vi "子界面-查看某框-不显示界面.vi"(0 "框号":dbl format="%#_13g", 1 "框组":T3(array[cluster]), 2 "临界Z值":i32, 3 "反射图原始路径":path, 4 "临界面积百分比值":dbl, 5 "预先配置的灰度阈值":dbl, 6 "穿透图原始路径":path, 7 "部位信息":string[](array[string])=["", "34.500000", "32.500000", "1121", "34", "54.955926", "分层类", "不合格", ""], 12 "产品规格":cluster{"产品长度（周长）（mm）":dbl, "产品宽度（母线长）（mm）":dbl}) -> (14 "弥散类检测结果":string[][](table), 19 "分层类检测结果":string[][](table))   [LabVIEW 2018]
uses:
  <vilib>/vision/NI_Vision_Development_Module.lvlib
panel:
  out "弥散和分层临界灰度值":i32
  out "弥散缺陷个数":i32
  out "分层缺陷个数":i32
  out "合格？ 弥散类":string="fencengThreshold"
  out "合格？分层类":string="fencengThreshold"
  out "?":T1(plugin-control)
  out "Threshold Image":T1(plugin-control)
  out "Threshold Image":T1(plugin-control)
  out "Threshold Image":T1(plugin-control)
  in  "Tab Control":T2
  out "穿透ROI":T1(plugin-control)
  out "Threshold Image":T1(plugin-control)
  out "?":T1(plugin-control)
  out "?":T1(plugin-control)
  out "Threshold Image":T1(plugin-control)
  out "Threshold Image":T1(plugin-control)
  out "弥散测量结果":dbl[][](array[numeric]) format="%.2f"
  in  "分隔符（'\\'代码显示）":string="\t"
  in  "格式字符串":string="%f"
  out "面积 (pixels)":i32
  in  "格式字符串 2":string="%f"
  in  "分隔符（'\\'代码显示）":string="\t"
  out "分层测量结果":dbl[][](array[numeric]) format="%.2f"
  out "缺陷分类的临界值":sgl format="%#.3f"
  # "所选区域信息"
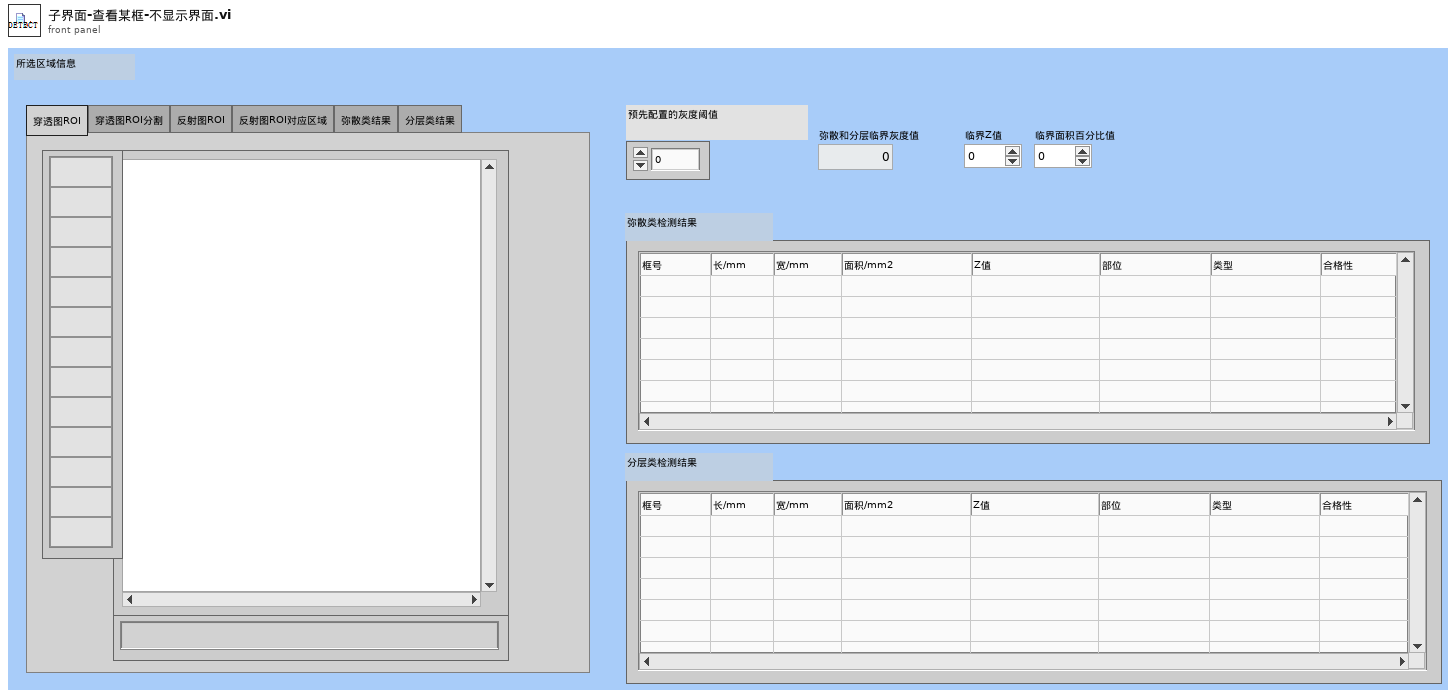
[diagram p1: front panel]
types:
  T1 = typedef "IMAQ Image.ctl" = refnum<image>
  T2 = typedef "控件 1.ctl" = enum32{"穿透图ROI", "穿透图ROI分割", "反射图ROI", "反射图ROI对应区域", "弥散类结果", "分层类结果"}
  T3 = cluster{"Global Rectangle":i32[], "Contours":cluster{"Contour Type":u32, "ROI Type":u32, "Points":i32[]}[]}[]
  T4 = typedef "Image Type" = u32
  T5 = typedef "Particle Parameters" = i32
  T6 = cluster{"Measurement Parameter":T5, "Range Lower Value":dbl, "Range Upper Value":dbl, "Range":bool, "Measurement Type":bool}[]
  T7 = cluster{"Global Rectangle":i32[], "Contours":cluster{"Contour Type":u32, "ROI Type":u32, "Points":i32[]}[]}
  T8 = cluster{"histogram":u32[], "Minimal Value":sgl, "Maximal Value":sgl, "Starting Value":sgl, "Interval Width":sgl, "Mean Value":sgl, "Standard  Variation":sgl, "Area (pixels)":i32}
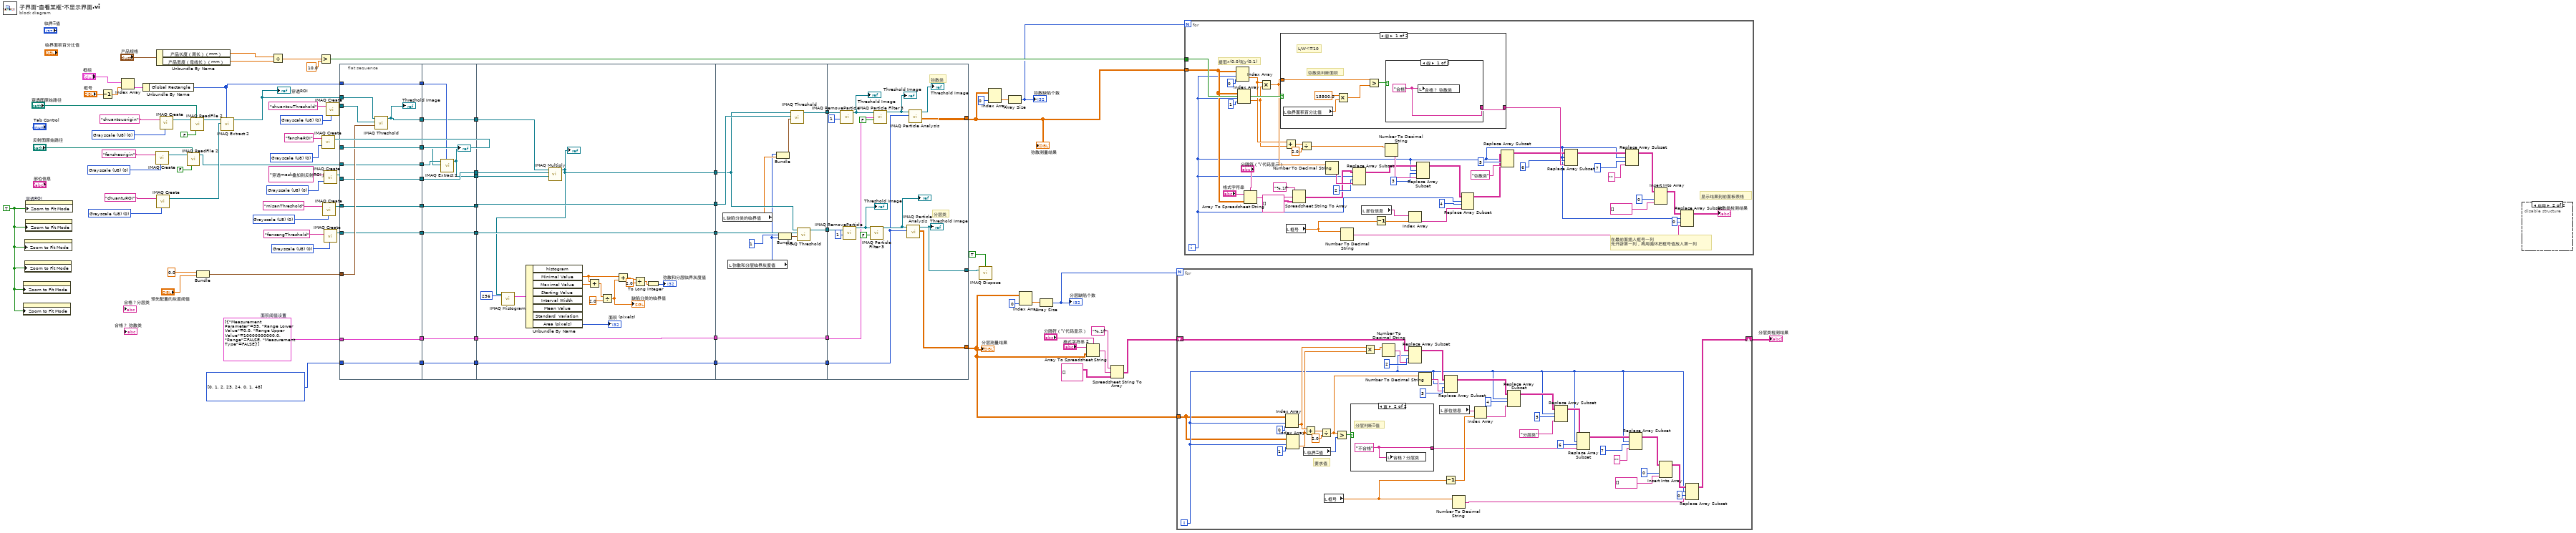
[diagram p0: block diagram]
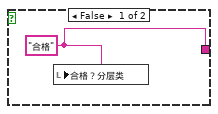
[diagram p2: hidden frame]
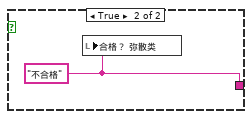
[diagram p3: hidden frame]
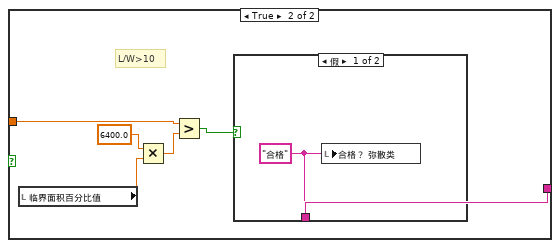
[diagram p4: hidden frame]
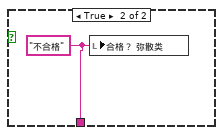
[diagram p5: hidden frame]
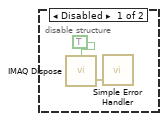
[diagram p6: hidden frame]
diagram:
  w55 = T4 0 items=["Grayscale (U8)", "Grayscale (I16)", "Grayscale (SGL)", "Complex (CSG)", "RGB (U32)", "HSL (U32)", "RGB (U64)", "Grayscale (U16)"] ("Image Type")
  w56 = T4 0 items=["Grayscale (U8)", "Grayscale (I16)", "Grayscale (SGL)", "Complex (CSG)", "RGB (U32)", "HSL (U32)", "RGB (U64)", "Grayscale (U16)"] ("Image Type")
  w57 = T4 0 items=["Grayscale (U8)", "Grayscale (I16)", "Grayscale (SGL)", "Complex (CSG)", "RGB (U32)", "HSL (U32)", "RGB (U64)", "Grayscale (U16)"] ("Image Type")
  w61 = T4 0 items=["Grayscale (U8)", "Grayscale (I16)", "Grayscale (SGL)", "Complex (CSG)", "RGB (U32)", "HSL (U32)", "RGB (U64)", "Grayscale (U16)"] ("Image Type")
  w65 = T4 0 items=["Grayscale (U8)", "Grayscale (I16)", "Grayscale (SGL)", "Complex (CSG)", "RGB (U32)", "HSL (U32)", "RGB (U64)", "Grayscale (U16)"] ("Image Type")
  w14 = i32[] [0, 1, 2, 23, 24, 0, 1, 48] items=["Bounding Rect Width", "Bounding Rect Height", "Area"] ("Pixel Measurements")
  w19 = T6 [{"Measurement Parameter"=35, "Range Lower Value"=0.0, "Range Upper Value"=10000000000.0, "Range"=FALSE, "Measurement Type"=FALSE}]  # 面积阈值设置
  w78 = T4 0 items=["Grayscale (U8)", "Grayscale (I16)", "Grayscale (SGL)", "Complex (CSG)", "RGB (U32)", "HSL (U32)", "RGB (U64)", "Grayscale (U16)"] ("Image Type")
  w48 = T4 0 items=["Grayscale (U8)", "Grayscale (I16)", "Grayscale (SGL)", "Complex (CSG)", "RGB (U32)", "HSL (U32)", "RGB (U64)", "Grayscale (U16)"] ("Image Type")
  w82 = T4 0 items=["Grayscale (U8)", "Grayscale (I16)", "Grayscale (SGL)", "Complex (CSG)", "RGB (U32)", "HSL (U32)", "RGB (U64)", "Grayscale (U16)"] ("Image Type")
  w90 = TRUE ("Zoom to Fit Mode")
  n1 = property class="ImageControl"("Zoom to Fit Mode"=w90) -> ()  [unwired: 2 in, 2 out]
  n2 = property class="ImageControl"("Zoom to Fit Mode"=w90) -> ()  [unwired: 2 in, 2 out]
  n3 = property class="ImageControl"("Zoom to Fit Mode"=w90) -> ()  [unwired: 2 in, 2 out]
  n4 = property class="ImageControl"("Zoom to Fit Mode"=w90) -> ()  [unwired: 2 in, 2 out]
  n5 = property class="ImageControl"("Zoom to Fit Mode"=w90) -> ()  [unwired: 2 in, 2 out]
  n6 = property on="穿透ROI" class="ImageControl"("Zoom to Fit Mode"=w90) -> ()  [unwired: 2 in, 2 out]
  n7 = Decrement(x="框号") -> (x-1=w84:dbl)
  n8 = Index Array(array="框组", index=w84) -> (element=w85:T7)
  n9 = Unbundle By Name(w85) -> ("Global Rectangle"=w47:i32[])
  n10 = call "IMAQ Create"("Image Name"="fansheorigin", "Image Type"=w61) -> ("New Image"=w60:T1)  [unwired: 3 in, 1 out]
  n11 = call "IMAQ Create"("Image Name"="chuantuROI", "Image Type"=w65) -> ("New Image"=w64:T1)  [unwired: 3 in, 1 out]
  n12 = Unbundle By Name("产品规格") -> ("产品长度（周长）（mm）"=w73:dbl, "产品宽度（母线长）（mm）"=w72:dbl)
  n13 = call "IMAQ Create"("Image Name"="chuantouorigin", "Image Type"=w82) -> ("New Image"=w67:T1)  [unwired: 3 in, 1 out]
  n14 = call "IMAQ ReadFile 2"("Use File Path Image Type"=FALSE, "File Path"="反射图原始路径", "Image"=w60) -> ("Image Out"=w43:T1)  [unwired: 4 in, 4 out]
  n15 = call "IMAQ ReadFile 2"("Use File Path Image Type"=FALSE, "File Path"="穿透图原始路径", "Image"=w67) -> ("Image Out"=w68:T1)  [unwired: 4 in, 4 out]
  n16 = Bundle(0.0, "预先配置的灰度阈值"="预先配置的灰度阈值") -> (w9:cluster{dbl, "预先配置的灰度阈值":dbl})  [unwired: 1 in]
  n17 = call "IMAQ Extract 2"("Optional Rectangle"=w47, "Image Dst"=w64, "Image Src"=w68) -> ("Image Dst Out"=w45:T1)  [unwired: 7 in, 1 out]
  "穿透ROI" <- w45
  n18 = Divide(x=w73, y=w72) -> (x/y=w76:dbl)
  n19 = Greater?(x=w76, y=10.0) -> (0:w71:bool)
  n20 = call "IMAQ Create"("Image Name"="fansheROI", "Image Type"=w48) -> ("New Image"=w44:T1)  [unwired: 3 in, 1 out]
  n21 = call "IMAQ Create"("Image Name"="misanThreshold", "Image Type"=w55) -> ("New Image"=w30:T1)  [unwired: 3 in, 1 out]
  n22 = call "IMAQ Create"("Image Name"="穿透mask叠加到反射ROI上", "Image Type"=w78) -> ("New Image"=w38:T1)  [unwired: 3 in, 1 out]
  n23 = call "IMAQ Create"("Image Name"="fencengThreshold", "Image Type"=w56) -> ("New Image"=w28:T1)  [unwired: 3 in, 1 out]
  n24 = call "IMAQ Create"("Image Name"="chuantouThreshold", "Image Type"=w57) -> ("New Image"=w46:T1)  [unwired: 3 in, 1 out]
  n25 = flat-sequence {
    tunnel: w47 -> [w102]
    tunnel: w46 -> [w101]
    tunnel: w45 -> [w100]
    tunnel: w9 -> [w99]
    tunnel: w44 -> [w98]
    tunnel: w43 -> [w97]
    tunnel: [w102] -> w42
    tunnel: [w98] -> w41
    tunnel: [w97] -> w40
    tunnel: [w96] -> w39
    tunnel: w38 -> [w96]
    tunnel: [w95] -> w35
    tunnel: w30 -> [w94]
    tunnel: [w94] -> w32
    tunnel: [w93] -> w29
    tunnel: w28 -> [w93]
    tunnel: [w92] -> w20
    tunnel: w19 -> [w92]
    tunnel: [w91] -> w15
    tunnel: w14 -> [w91]
    tunnel: w42 -> [w112]
    tunnel: w41 -> [w103]
    tunnel: w40 -> [w104]
    tunnel: w39 -> [w111]
    tunnel: [w111] -> w37
    tunnel: [w110] -> w36
    tunnel: w35 -> [w110]
    tunnel: [w109] -> w34
    tunnel: w32 -> [w108]
    tunnel: [w108] -> w31
    tunnel: w29 -> [w107]
    tunnel: [w107] -> w27
    tunnel: w20 -> [w106]
    tunnel: [w106] -> w18
    tunnel: w15 -> [w105]
    tunnel: [w105] -> w13
    tunnel: w37 -> [w132]
    tunnel: w36 -> [w131]
    tunnel: w34 -> [w130]
    tunnel: [w129] -> w33
    tunnel: w31 -> [w129]
    tunnel: w27 -> [w128]
    tunnel: [w128] -> w26
    tunnel: [w123] -> w25
    tunnel: w18 -> [w122]
    tunnel: [w122] -> w17
    tunnel: w13 -> [w121]
    tunnel: [w121] -> w12
    tunnel: w33 -> [w144]
    tunnel: w26 -> [w143]
    tunnel: w25 -> [w142]
    tunnel: [w141] -> w22
    tunnel: [w140] -> w21
    tunnel: w17 -> [w139]
    tunnel: [w139] -> w16
    tunnel: w12 -> [w138]
    tunnel: [w138] -> w11
    tunnel: [w155] -> w24
    tunnel: [w150] -> w3
    tunnel: [w149] -> w23
    tunnel: w22 -> [w148]
    tunnel: w21 -> [w147]
    tunnel: w16 -> [w146]
    tunnel: w11 -> [w145]
    frame #0 {
      n26 = call "IMAQ Threshold"("Range"=w99, "Image Dst"=w101, "Image Src"=w100) -> ("Image Dst Out"=w95:T1)  [unwired: 3 in, 5 out]
      "Threshold Image" <- w95
    }
    frame #1 {
      n27 = call "IMAQ Extract 2"("Optional Rectangle"=w112, "Image Dst"=w103, "Image Src"=w104) -> ("Image Dst Out"=w109:T1)  [unwired: 7 in, 1 out]
      "?" <- w109
    }
    frame #2 {
      n28 = call "IMAQ Multiply"("Image Src A"=w131, "Image Dst"=w132, "Image Src B"=w130) -> ("Image Dst Out"=w123:T1)  [unwired: 4 in, 1 out]
      "?" <- w123
      n29 = call "IMAQ Histogram"("Number of Classes"=256, "Image"=w123) -> ("Histogram Report"=w126:T8)  [unwired: 8 in, 1 out]
      n30 = Unbundle By Name(w126) -> ("Minimal Value"=w113:sgl, "Maximal Value"=w115:sgl, "Area (pixels)"=→"面积 (pixels)":i32)  [unwired: 5 out]
      n31 = Add(x=w113, y=w115) -> (x+y=w114:sgl)
      n32 = Divide(x=w114, y=sgl 2.0) -> (x/y=w116:sgl)
      "缺陷分类的临界值" <- w116
      n33 = Add(x=w113, y=w116) -> (x+y=w120:sgl)
      n34 = Divide(x=w120, y=sgl 2.0) -> (x/y=w118:sgl)
      n35 = To Long Integer(number=w118) -> (32bit integer=→"弥散和分层临界灰度值":i32)
    }
    frame #3 {
      n36 = local read "缺陷分类的临界值"() -> (w137:sgl)
      n37 = local read "弥散和分层临界灰度值"() -> (w135:i32)
      n38 = Bundle("弥散和分层临界灰度值"=w135, "缺陷分类的临界值"=w137) -> (w136:cluster{"弥散和分层临界灰度值":i32, "缺陷分类的临界值":sgl})  [unwired: 1 in]
      n39 = Bundle(1, "弥散和分层临界灰度值"=w135) -> (w133:cluster{i32, "弥散和分层临界灰度值":i32})  [unwired: 1 in]
      n40 = call "IMAQ Threshold"("Range"=w136, "Image Dst"=w144, "Image Src"=w142) -> ("Image Dst Out"=w140:T1)  [unwired: 3 in, 5 out]
      n41 = call "IMAQ Threshold"("Range"=w133, "Image Dst"=w143, "Image Src"=w142) -> ("Image Dst Out"=w141:T1)  [unwired: 3 in, 5 out]
    }
    frame #4 {
      # "分层类"
      # "弥散类"
      n42 = call "IMAQ RemoveParticle"("Number of Erosion"=1, "Image Src"=w147) -> ("Image Dst Out"=w158:T1)  [unwired: 8 in, 1 out]
      "Threshold Image" <- w158
      n43 = call "IMAQ RemoveParticle"("Number of Erosion"=1, "Image Src"=w148) -> ("Image Dst Out"=w153:T1)  [unwired: 8 in, 1 out]
      "Threshold Image" <- w153
      n44 = call "IMAQ Particle Filter 3"("Image Src"=w153, "Keep/Remove Particles (F)"=FALSE) -> ("Image Dst Out"=w154:T1)  [unwired: 11 in, 2 out]
      "?" <- w154
      n45 = call "IMAQ Particle Filter 3"("Image Src"=w158, "Selection Values"=w146, "Keep/Remove Particles (F)"=FALSE) -> ("Image Dst Out"=w159:T1)  [unwired: 10 in, 2 out]
      "Threshold Image" <- w159
      n46 = call "IMAQ Particle Analysis"("Pixel Measurements"=w145, "Image"=w154) -> ("Particle Measurements (Pixels)"=w150:dbl[][], "Image Out (duplicate)"=w149:T1)  [unwired: 4 in, 4 out]
      "Threshold Image" <- w149
      n47 = call "IMAQ Particle Analysis"("Pixel Measurements"=w145, "Image"=w159) -> ("Particle Measurements (Real-World)"=w155:dbl[][], "Image Out (duplicate)"=→"Threshold Image":T1)  [unwired: 4 in, 4 out]
    }
  }
  n48 = call "IMAQ Dispose"("All Images? (No)"=TRUE, "Image"=w23) -> ()  [unwired: 4 in, 1 out]
  n49 = Index Array(array=w24, index (col)=0 ("禁用的索引 (列)")) -> (element=w51:dbl[])  [unwired: 1 in]
  n50 = Array Size(array=w51) -> (size(s)=w70:i32)
  "弥散缺陷个数" <- w70
  n51 = Index Array(array=w3, index (col)=0 ("禁用的索引 (列)")) -> (element=w53:dbl[])  [unwired: 1 in]
  n52 = Array Size(array=w53) -> (size(s)=w10:i32)
  "分层缺陷个数" <- w10
  n53 = Array To Spreadsheet String(delimiter (Tab)="分隔符（'\\'代码显示）", array=w3, 3:"格式字符串 2") -> (spreadsheet string=w6:string)
  n54 = Spreadsheet String To Array(format string="%.1f", spreadsheet string=w6, array type (2D Dbl)=string[][] [] ("Array")) -> (array=w2:string[][])  [unwired: 1 in]
  n55 = for {
    N: w10 -> [_]
    tunnel: w3 -> [w164]
    shift-right: [w161] -> w1
    shift-left: w2 -> [w162]
    i -> [w167]
    # "要求值"
    n56 = Index Array(array=w164, index (row)=w167, index (col)=0 ("禁用的索引 (列)")) -> (element=w180:dbl)
    n57 = Index Array(array=w164, index (row)=w167, index (col)=1 ("禁用的索引 (列)")) -> (element=w179:dbl)
    n58 = local read "临界Z值"() -> (w163:i32)
    n59 = Add(x=w180, y=w179) -> (x+y=w199:dbl)
    n60 = Divide(x=w199, y=2.0) -> (x/y=w193:dbl)
    n61 = local read "框号"() -> (w165:dbl)
    n62 = Greater?(x=w193, y=w163) -> (0:w200:bool)
    n63 = case shown="真" w200 {
      tunnel: [w201 w202] -> w173
      frame False {
        w201 = "合格" ("合格？")
        n64 = local write "合格？分层类"(w201) -> ()
      }
      frame True {
        w202 = "不合格" ("合格？")
        # "分层判断Z值"
        n65 = local write "合格？分层类"(w202) -> ()
      }
    }
    n66 = Multiply(x=w180, y=w179) -> (x*y=w191:dbl)
    n67 = Number To Decimal String(number=w191) -> (decimal integer string=w178:string)  [unwired: 1 in]
    n68 = Replace Array Subset(array=w162, new element=w178, index (row)=w167, index (col)=2 ("禁用的索引 (列)")) -> (w187:string[][])
    n69 = Number To Decimal String(number=w193) -> (decimal integer string=w177:string)  [unwired: 1 in]
    n70 = local read "部位信息"() -> (w184:string[])
    n71 = Decrement(x=w165) -> (x-1=w183:dbl)
    n72 = Replace Array Subset(array=w187, new element=w177, index (row)=w167, index (col)=3 ("禁用的索引 (列)")) -> (w182:string[][])
    n73 = Number To Decimal String(number=w165) -> (decimal integer string=w166:string)  [unwired: 1 in]
    n74 = Index Array(array=w184, index=w183) -> (element=w176:string)
    n75 = Replace Array Subset(array=w182, new element=w176, index (row)=w167, index (col)=4 ("禁用的索引 (列)")) -> (w181:string[][])
    n76 = Replace Array Subset(array=w181, new element="分层类" ("新元素/子数组"), index (row)=w167, index (col)=5 ("禁用的索引 (列)")) -> (w186:string[][])
    n77 = Replace Array Subset(array=w186, new element=w173, index (row)=w167, index (col)=6 ("禁用的索引 (列)")) -> (w189:string[][])
    n78 = Replace Array Subset(array=w189, new element="" ("新元素/子数组"), index (row)=w167, index (col)=7 ("禁用的索引 (列)")) -> (w168:string[][])
    n79 = Insert Into Array(array=w168, index (col)=0 ("禁用的索引 (列)"), new element=string[] [] ("新元素/子数组")) -> (w170:string[][])  [unwired: 1 in]
    n80 = Replace Array Subset(array=w170, new element=w166, index (row)=w167, index (col)=0 ("禁用的索引 (列)")) -> (w161:string[][])
  }
  "分层类检测结果" <- w1
  n81 = for {
    N: w70 -> [_]
    tunnel: w71 -> [w246]
    tunnel: w24 -> [w245]
    i -> [w206]
    # "在最前面插入框号一列\n先开辟第一列，再用循环把框号值放入第一列"
    # "提取x(0,0)和y(0,1)"
    # "显示结果到前面板表格"
    n82 = Index Array(array=w245, index (row)=w206, index (col)=0 ("禁用的索引 (列)")) -> (element=w229:dbl)
    n83 = Index Array(array=w245, index (row)=w206, index (col)=1 ("禁用的索引 (列)")) -> (element=w228:dbl)
    n84 = Array To Spreadsheet String(delimiter (Tab)="分隔符（'\\'代码显示）", array=w245, 3:"格式字符串") -> (spreadsheet string=w243:string)
    n85 = Multiply(x=w229, y=w228) -> (x*y=w232:dbl)
    n86 = case shown="假" w246 {
      tunnel: w232 -> [w252 w260]
      tunnel: [w250 w258] -> w244
      frame False {
        # "弥散类判断面积"
        # "L/W<=10"
        n87 = local read "临界面积百分比值"() -> (w247:dbl)
        n88 = Multiply(x=15500.0, y=w247) -> (x*y=w248:dbl)
        n89 = Greater?(x=w252, y=w248) -> (0:w251:bool)
        n90 = case shown="假" w251 {
          tunnel: [w253 w254] -> w250
          frame False {
            w253 = "合格" ("合格？")
            n91 = local write "合格？ 弥散类"(w253) -> ()
          }
          frame True {
            w254 = "不合格" ("合格？")
            n92 = local write "合格？ 弥散类"(w254) -> ()
          }
        }
      }
      frame True {
        # "L/W>10"
        n93 = local read "临界面积百分比值"() -> (w255:dbl)
        n94 = Multiply(x=6400.0 ("y"), y=w255) -> (x*y=w257:dbl)
        n95 = Greater?(x=w260, y=w257) -> (0:w259:bool)
        n96 = case shown="假" w259 {
          tunnel: [w261 w262] -> w258
          frame False {
            w261 = "合格" ("合格？")
            n97 = local write "合格？ 弥散类"(w261) -> ()
          }
          frame True {
            w262 = "不合格" ("合格？")
            n98 = local write "合格？ 弥散类"(w262) -> ()
          }
        }
      }
    }
    n99 = Add(x=w229, y=w228) -> (x+y=w231:dbl)
    n100 = local read "框号"() -> (w210:dbl)
    n101 = Spreadsheet String To Array(format string="%.1f", spreadsheet string=w243, array type (2D Dbl)=string[][] [] ("Array")) -> (array=w220:string[][])  [unwired: 1 in]
    n102 = Divide(x=w231, y=2.0) -> (x/y=w225:dbl)
    n103 = Number To Decimal String(number=w232) -> (decimal integer string=w234:string)  [unwired: 1 in]
    n104 = Number To Decimal String(number=w210) -> (decimal integer string=w204:string)  [unwired: 1 in]
    n105 = Replace Array Subset(array=w220, new element=w234, index (row)=w206, index (col)=2 ("禁用的索引 (列)")) -> (w219:string[][])
    n106 = local read "部位信息"() -> (w215:string[])
    n107 = Decrement(x=w210) -> (x-1=w214:dbl)
    n108 = Number To Decimal String(number=w225) -> (decimal integer string=w227:string)  [unwired: 1 in]
    n109 = Index Array(array=w215, index=w214) -> (element=w213:string)
    n110 = Replace Array Subset(array=w219, new element=w227, index (row)=w206, index (col)=3 ("禁用的索引 (列)")) -> (w212:string[][])
    n111 = Replace Array Subset(array=w212, new element=w213, index (row)=w206, index (col)=4 ("禁用的索引 (列)")) -> (w211:string[][])
    n112 = Replace Array Subset(array=w211, new element="弥散类" ("新元素/子数组"), index (row)=w206, index (col)=5 ("禁用的索引 (列)")) -> (w218:string[][])
    n113 = Replace Array Subset(array=w218, new element=w244, index (row)=w206, index (col)=6 ("禁用的索引 (列)")) -> (w217:string[][])
    n114 = Replace Array Subset(array=w217, new element="" ("新元素/子数组"), index (row)=w206, index (col)=7 ("禁用的索引 (列)")) -> (w209:string[][])
    n115 = Insert Into Array(array=w209, index (col)=0 ("禁用的索引 (列)"), new element=string[] [] ("新元素/子数组")) -> (w207:string[][])  [unwired: 1 in]
    n116 = Replace Array Subset(array=w207, new element=w204, index (row)=w206, index (col)=0 ("禁用的索引 (列)")) -> (→"弥散类检测结果":string[][])
  }
  n117 = disable-structure shown="启用" {
    frame Disabled {
      n118 = call "IMAQ Dispose"("All Images? (No)"=TRUE) -> ("error out"=w264:errorcluster)  [unwired: 5 in]
      n119 = call <vilib>:"Simple Error Handler.vi"("error in (no error)"=w264) -> ()  [unwired: 4 in, 5 out]
    }
    frame Enabled {
    }
  }
  "分层测量结果" <- w3
  "弥散测量结果" <- w24
